vi "4000 Compatible.vi"() -> ()   [LabVIEW 2012]
panel:
  out "4000 compatible?":bool=TRUE
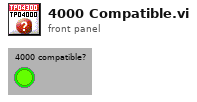
[diagram p1: front panel]
diagram:
